vi "GetFileFlowScript.vi"(8 "error in (no error)":errorcluster) -> (0 "error out":errorcluster, 2 "found":bool, 3 "Fileflow script":string[](array[string]))   [LabVIEW 2017, in "FileFlow.lvlib"]
uses:
  <vilib>/addons/InsightCM/Devices/Shared/Common/FileFlow/FileFlow.lvlib
  <vilib>/addons/PointValueMap/subVIs/Point_Read_variant.vi
  <vilib>/addons/InsightCM/Utilities/GlobalConfiguration/GlobalConfiguration.lvlib
  <vilib>/addons/PointValueMap/PointValueMap.lvlib
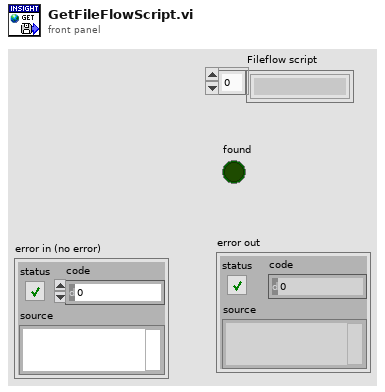
[diagram p1: front panel]
types:
  T1 = typedef "PointValueMap.lvlib/PointMap.ctl" = refnum<data-value>
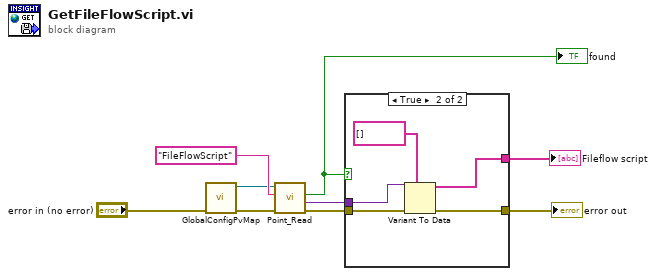
[diagram p0: block diagram]
diagram:
  n1 = call <vilib>:"GlobalConfigPvMap.vi"("error in (no error)"="error in (no error)") -> ("error out"=w8:errorcluster, "global configuration map"=w7:T1)  [unwired: 9 in]
  n2 = call-poly <vilib>:"Point_Read.vi"("Error In"=w8, "Tag"="FileFlowScript" ("Name"), "Map"=w7) -> ("Error Out"=w5:errorcluster, "Value"=w3:variant, "Found?"=w1:bool)  [unwired: 3 in, 3 out]
  "found" <- w1
  n3 = case shown="True" w1 {
    tunnel: w5 -> [w10 w14]
    tunnel: [w10 w13] -> w4
    tunnel: w3 -> [_ w12]
    tunnel: [_ w11] -> w2
    frame False {
    }
    frame True {
      n4 = Variant To Data(error in=w14, type=string[] [] ("DataFlow"), Variant=w12) -> (data=w11:string[], error out=w13:errorcluster)
    }
  }
  "error out" <- w4
  "Fileflow script" <- w2
